vi "PluginTypeArray.vi"(8 "ErrorArray Out in":errorcluster[](array[cluster]), 10 "INIFilePaths":path[](array[path]), 11 "section":string) -> (0 "ErrorArray Out out":errorcluster[](array[cluster]), 2 "PluginTypes":string[](array[string]), 3 "IniFilePaths":path[](array[path]))   [LabVIEW 2014, in "Ini_lib.lvlib"]
uses:
  <vilib>/Utility/config.llb/Read Key (String).vi
  <vilib>/Utility/error.llb/Error Cluster From Error Code.vi
  <vilib>/ErrorRing/Error Ring.xnode
  Ini_lib.lvlib
  <vilib>/Utility/config.llb/NI_LVConfig.lvlib
  <userlib>/NIST/NISTErrorLib/NISTErrorLib.lvlib
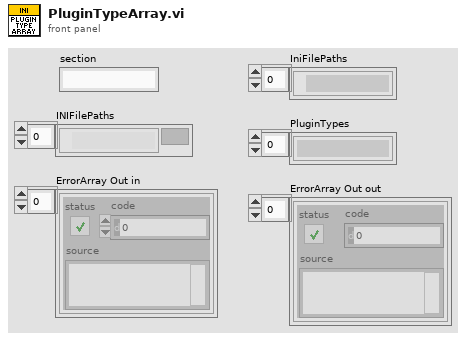
[diagram p1: front panel]
types:
  T1 = typedef "NI_LVConfig.lvlib/Config Data RefNum.ctl" = refnum<k1>
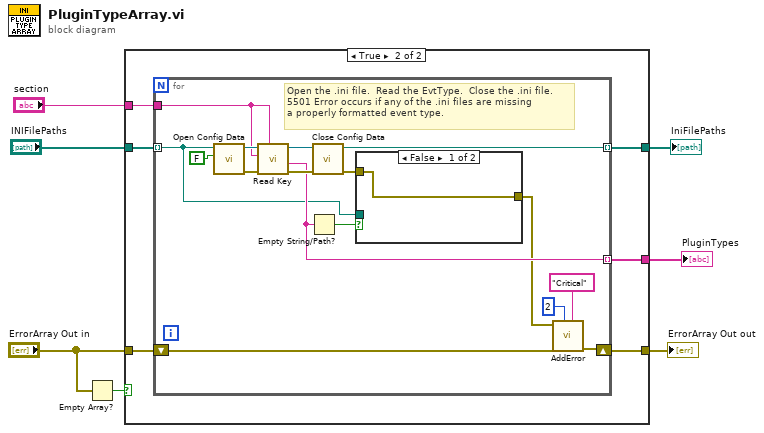
[diagram p0: block diagram]
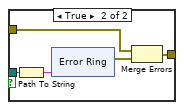
[diagram p3: hidden frame]
diagram:
  n1 = Empty Array?(array="ErrorArray Out in") -> (empty?=w2:bool)
  n2 = case shown="True" w2 {
    tunnel: "section" -> [_ w15]
    tunnel: "ErrorArray Out in" -> [w8 w14]
    tunnel: "INIFilePaths" -> [w9 w13]
    tunnel: [w9 w12] -> w5
    tunnel: [w8 w11] -> w4
    tunnel: [_ w10] -> w3
    frame False {
    }
    frame True {
      n3 = for {
        tunnel: w13 -> [w16] mode=indexing
        tunnel: [w25] -> w10 mode=indexing
        tunnel: [w26] -> w12 mode=indexing
        shift-right: [w19] -> w11
        shift-left: w14 -> [w20]
        tunnel: w15 -> [w17]
        # "Open the .ini file.  Read the EvtType.  Close the .ini file.\n5501 Error occurs if any of the .ini files are missing\na properly formatted event type."
        n4 = call <vilib>:"Open Config Data.vi"("create file if necessary (T)"=FALSE, "configuration file path"=w16) -> ("error out"=w30:errorcluster, "refnum"=w29:T1)  [unwired: 7 in, 1 out]
        n5 = call-poly <vilib>:"Read Key.vi"("section"=w17, "error in (no error)"=w30, "key"=w17, "refnum"=w29) -> ("error out"=w27:errorcluster, "value"=w25:string, "refnum out"=w28:T1)  [unwired: 4 in, 1 out]
        n6 = Empty String/Path?(string/path=w25) -> (empty?=w24:bool)
        n7 = call <vilib>:"Close Config Data.vi"("error in (no error)"=w27, "refnum"=w28) -> ("error out"=w23:errorcluster, "file path"=w26:path)  [unwired: 8 in]
        n8 = case shown="False" w24 {
          tunnel: w23 -> [w32 w36]
          tunnel: [w32 w35] -> w18
          tunnel: w16 -> [_ w33]
          frame False {
          }
          frame True {
            n9 = Path To String(path=w33) -> (string=w34:string)
            n10 = xnode "Error Ring"("parameter 0"=w34) -> ("error out"=w37:errorcluster)
            n11 = Merge Errors(w36, w37) -> (w35:errorcluster)
          }
        }
        n12 = call <userlib>:"AddError.vi"("Severity"="Critical" ("String"), "Priority"=u8 2, "ErrorArray"=w20, "error in (no error)"=w18) -> ("ErrorArray"=w19:errorcluster[])  [unwired: 6 in, 1 out]
      }
    }
  }
  "IniFilePaths" <- w5
  "ErrorArray Out out" <- w4
  "PluginTypes" <- w3
